vi "example_3_3_a.vi"   [LabVIEW 2018]
panel:
  # "NOTE: remember plug the Led Analyser\nbefore run LabVIEW and to change the\nVISA resource name in the schematic,\notherwise the application will not work."
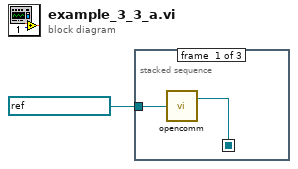
[diagram p0: block diagram]
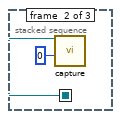
[diagram p2: hidden frame]
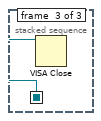
[diagram p3: hidden frame]
diagram:
  n1 = stacked-sequence {
    seq-local: [w2 _ _] -> [_ w4 w6]
    tunnel: refnum<visa-resource-name> "ASRL20::INSTR" -> [w3 _ _]
    frame #0 {
      n2 = call "opencomm.vi"("VISA resource name"=w3) -> ("duplicate VISA resource name"=w2:refnum<visa-resource-name>)  [unwired: 1 out]
    }
    frame #1 {
      n3 = call "capture.vi"("Capture Range"=0 ("Capture Type"), "VISA resource name"=w4) -> ()  [unwired: 2 in, 2 out]
    }
    frame #2 {
      n4 = VISA Close(VISA resource name=w6) -> ()  [unwired: 1 in, 1 out]
    }
  }
